vi "PH_Get6PInformation.panel.vi"(0 "object ref":refnum<vi>, 5 "error in (no error)":errorcluster) -> (19 "error out":errorcluster)   [LabVIEW 2014, in "PH_Get6PInformation.lvlib"]
doc: "By this VI infoamation about cams is indicated.\n\n\"EXIT\" closes the front panel (GUI), while \"Delete Instance\" disconnects and removes the instance from the PCS.\n\n\nLicense Agreement for this software:\n\nCopyright (C)\nGesellschaft für Schwerionenforschung, GSI\nPlanckstr. 1\n64291 Darmstadt\nGermany\n\nContact: D.Beck@gsi.de \n\nThis program is free software; you can redistribute it and/or modify it under the terms of the GNU General Public License as published by the Free Software Foundation; either version 2 of the license, or (at your option) any later version.\n\nThis program is distributed in the hope that it will be useful, but WITHOUT ANYW ARRANTY; without even the implied warranty of MERCHANTABILITY or FITNESS FOR A PARTICULAR PURPOSE. See the GNU General License for more details (http://www.gnu.org).\n\nGesellschaft für Schwerionenforschung, GSI\nPlanckstr. 1, 64291 Darmstadt, Germany\nFor all questions and ideas contact: M.Richter@gsi.de, H.Brand@gsi.de or D.Beck@gsi.de.\nLast update: 18-DEC-2002"
uses:
  PH_Get6PInformation.lvlib
  PH_Common/PH_Common.lvlib
  PH_GUI_Class/PH_GUI_Class.lvlib
panel:
  in  "Get Beckhoff Motion Parameters":bool
  in  "Get Sixpack Parameters":bool
  in  "PCS Motion List":i32(listbox)
  in  "Save Information":bool
  in  "Get Information":bool
  in  "Delete":bool
  # "PCS"
  # "3.40"
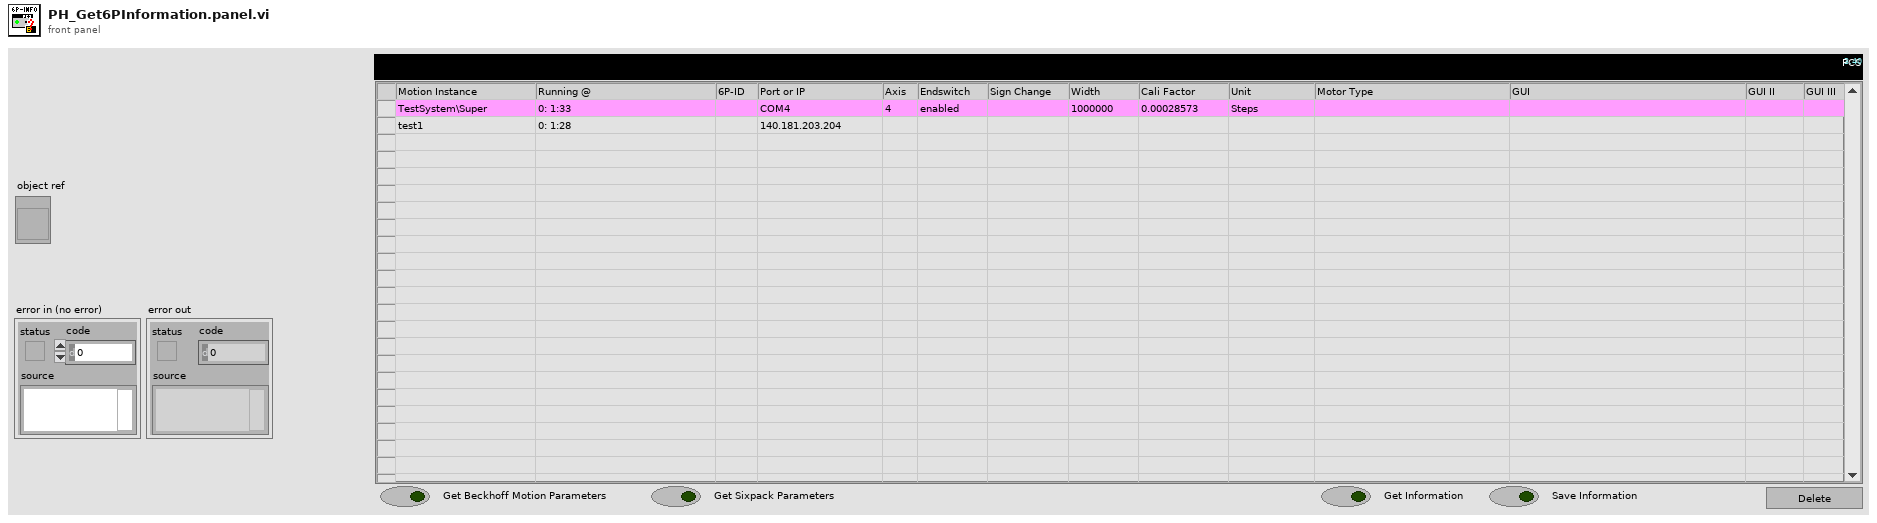
[diagram p1: front panel]
types:
  T1 = enum32{"Invalid", "Standard", "Closed", "Hidden", "Minimized", "Maximized"}
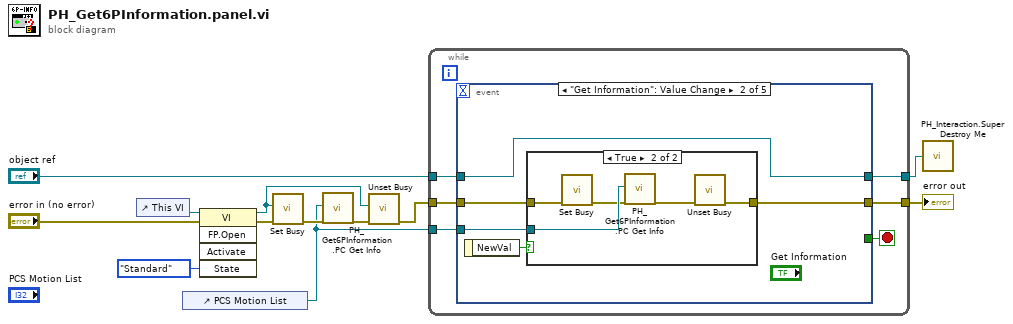
[diagram p0: block diagram]
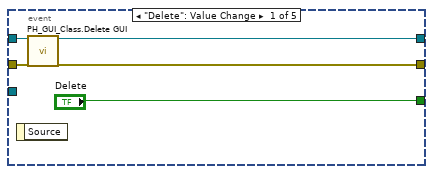
[diagram p2: hidden frame]
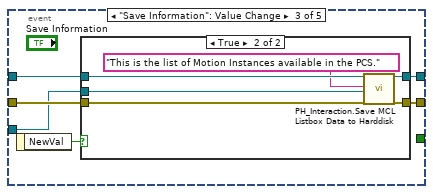
[diagram p4: hidden frame]
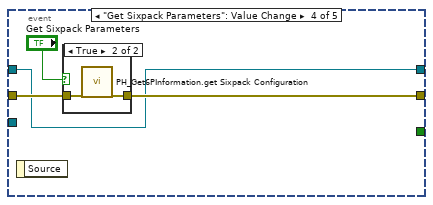
[diagram p6: hidden frame]
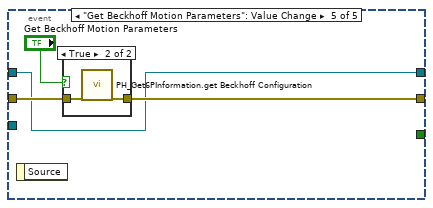
[diagram p8: hidden frame]
diagram:
  n1 = control-ref of="This VI"() -> (w8:refnum<vi>)
  n2 = control-ref of="PCS Motion List"() -> (w1:refnum<vi>)
  n3 = invoke class="VI" method="FP.Open"(reference=w8, error in="error in (no error)", "State"=T1."Standard") -> (reference out=w4:refnum<vi>, error out=w3:errorcluster)  [unwired: 2 in, 3 out]
  n4 = call <vilib>:"Set Busy.vi"("error in (no error)"=w3, "VI reference (current VI)"=w4) -> ("error out"=w6:errorcluster)  [unwired: 8 in, 1 out]
  n5 = call "PH_Get6PInformation.PC Get Info.vi"("PCS Motion List Ref"=w1, "error in"=w6) -> ("error out"=w5:errorcluster)  [unwired: 17 in]
  n6 = call <vilib>:"Unset Busy.vi"("error in (no error)"=w5, "VI reference (current VI)"=w4) -> ("error out"=w2:errorcluster)  [unwired: 9 in]
  n7 = while {
    tunnel: "object ref" -> [w17]
    tunnel: w2 -> [w16]
    tunnel: [w15] -> w12
    tunnel: w1 -> [w14]
    tunnel: [w13] -> w11
    stop <- w18 stop-if-true
    n8 = event shown="[1] \"Get Information\": Value Change" {
      selector: _ -> [_ _ _ _ _]
      dyn-events: _ -> [_ _ _ _ _]
      timeout: _ -> [_ _ _ _ _]
      tunnel: ["Delete" _ _ _ _] -> w18
      tunnel: w17 -> [w21 w24 w38 w49 w57]
      tunnel: w16 -> [w23 w28 w40 w51 w58]
      tunnel: [w19 w27 w39 w52 w59] -> w15
      tunnel: w14 -> [_ w25 w36 _ _]
      tunnel: [w20 w24 w35 w49 w57] -> w13
      event "Delete": Value Change {
        n9 = event-data() -> ()  [unwired: 1 in, 1 out]
        n10 = call "PH_GUI_Class.Delete GUI.vi"("VI in"=w21, "error in (no error)"=w23) -> ("VI out"=w20:refnum<vi>, "error out"=w19:errorcluster)  [unwired: 16 in]
      }
      event "Get Information": Value Change {
        n11 = event-data() -> ("NewVal"=w26:bool)  [unwired: 1 in]
        n12 = case shown="True" w26 {
          tunnel: w28 -> [w29 w33]
          tunnel: [w29 w30] -> w27
          tunnel: w25 -> [_ w34]
          frame False {
          }
          frame True {
            n13 = call <vilib>:"Set Busy.vi"("error in (no error)"=w33) -> ("error out"=w32:errorcluster)  [unwired: 9 in, 1 out]
            n14 = call "PH_Get6PInformation.PC Get Info.vi"("PCS Motion List Ref"=w34, "error in"=w32) -> ("error out"=w31:errorcluster)  [unwired: 17 in]
            n15 = call <vilib>:"Unset Busy.vi"("error in (no error)"=w31) -> ("error out"=w30:errorcluster)  [unwired: 10 in]
          }
        }
      }
      event "Save Information": Value Change {
        n16 = event-data() -> ("NewVal"=w37:bool)  [unwired: 1 in]
        n17 = case shown="True" w37 {
          tunnel: w40 -> [w42 w44]
          tunnel: [w42 w48] -> w39
          tunnel: w38 -> [w41 w47]
          tunnel: w36 -> [_ w45]
          tunnel: [w41 w46] -> w35
          frame False {
          }
          frame True {
            n18 = call "PH_Interaction.Save MCL Listbox Data to Harddisk.vi"("VI in"=w47, "Headline"="This is the list of Motion Instances available in the PCS." ("string"), "MCL Listbox GUI Reference"=w45, "error in (no error)"=w44) -> ("VI out"=w46:refnum<vi>, "error out"=w48:errorcluster)  [unwired: 14 in]
          }
        }
      }
      event "Get Sixpack Parameters": Value Change {
        n19 = event-data() -> ()  [unwired: 1 in, 1 out]
        n20 = case shown="True" "Get Sixpack Parameters" {
          tunnel: [w53 w54] -> w52
          tunnel: w51 -> [w53 w55]
          frame False {
          }
          frame True {
            n21 = call "PH_Get6PInformation.get Sixpack Configuration.vi"("error in (no error)"=w55) -> ("error out"=w54:errorcluster)  [unwired: 18 in]
          }
        }
      }
      event "Get Beckhoff Motion Parameters": Value Change {
        n22 = event-data() -> ()  [unwired: 1 in, 1 out]
        n23 = case shown="True" "Get Beckhoff Motion Parameters" {
          tunnel: [w60 w61] -> w59
          tunnel: w58 -> [w60 w62]
          frame False {
          }
          frame True {
            n24 = call "PH_Get6PInformation.get Beckhoff Configuration.vi"("error in (no error)"=w62) -> ("error out"=w61:errorcluster)  [unwired: 18 in]
          }
        }
      }
    }
  }
  "error out" <- w12
  n25 = call "PH_Interaction.Super Destroy Me.vi"("i ref out"=w11) -> ()
